vi "Edit_Channel_Panel.vi"(0 "All Channel names":string[](array[string])=["30-10-03:New:Channel new5"], 9 "Result files to read":path[](array[path])) -> (3 "New Values Out":string[](array[string])=["Test data5"], 4 "New Chs Out":string[](array[string])=["30-10-03:New:Channel new5"], 6 "Cancel Out":bool, 8 "Edit Raw Data Header Info Out":bool, 10 "Plotted rows only?":bool, 13 "Edit Raw data files?":bool, 14 "Raw data files in Orig Positions?":bool, 15 "Mode":T1)   [LabVIEW 2010]
uses:
  Plotter_Mode.ctl
panel:
  in  "Select channel names":bool
  in  "Cancel":bool
  in  "Edit Raw data files":i32(listbox)
  in  "Columns to Output":i32[](listbox)
  in  "Edit Type":i32(listbox)
  in  "OK Button":bool
  in  "Add values to:":i32(listbox)=1
  in  "New Values In":string[](array[string])=["Value"]
  in  "New Chs In":string[](array[string])=["Channel Name"]
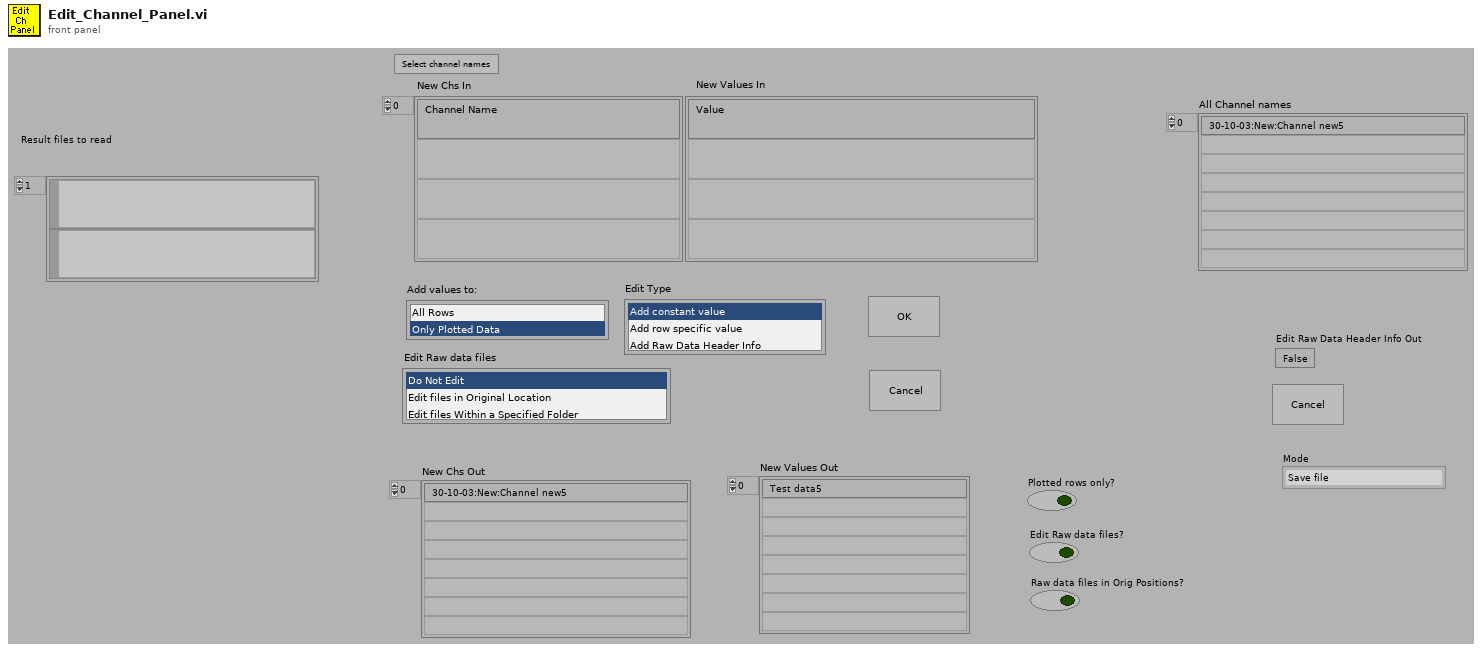
[diagram p1: front panel]
types:
  T1 = typedef "Plotter_Mode.ctl" = enum16{"Save file", "Delete unwanted rows", "Edit Values with constants", "Edit values per row", "Edit Raw Data file header", "Post Process Plotted Rows"}
  T2 = enum16{"Read Channels From File", "Read Channels from Server"}
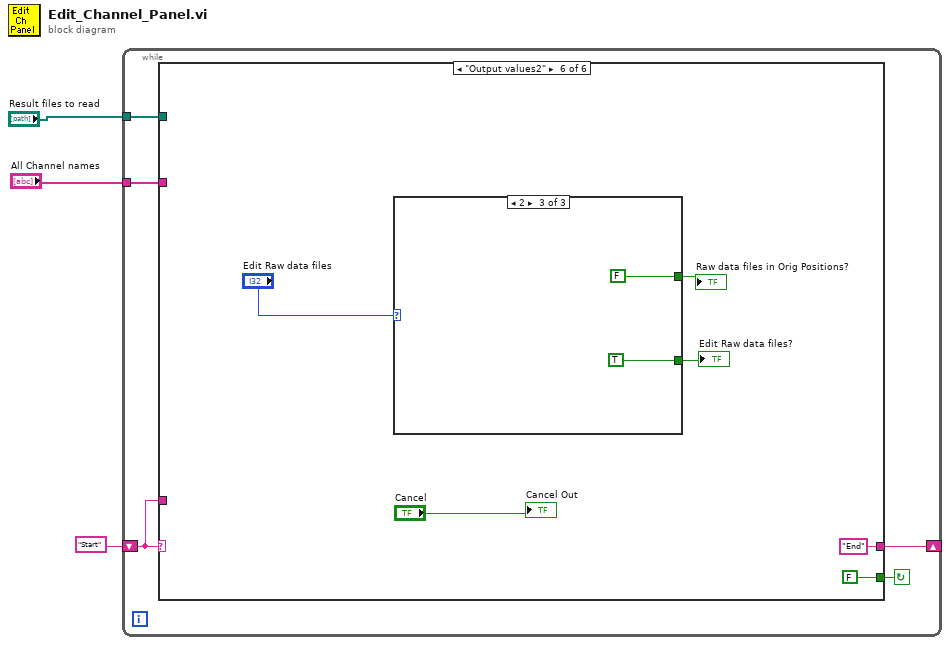
[diagram p0: block diagram]
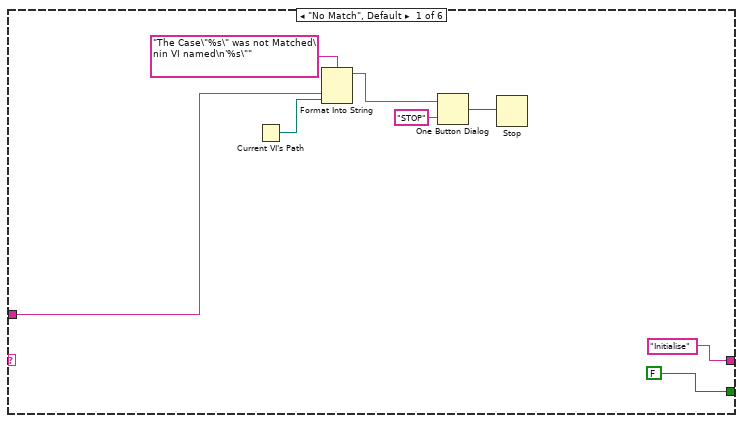
[diagram p2: hidden frame]
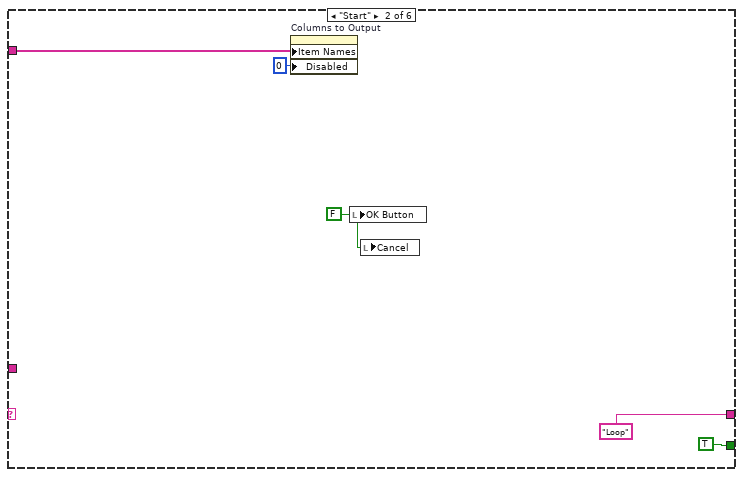
[diagram p3: hidden frame]
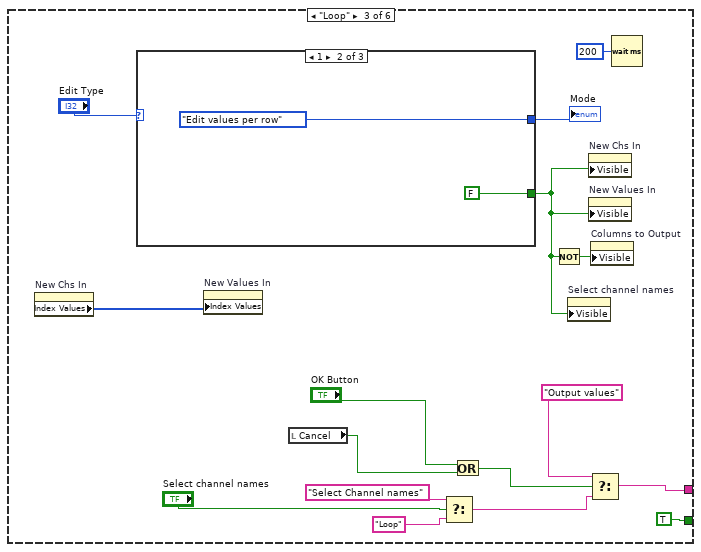
[diagram p4: hidden frame]
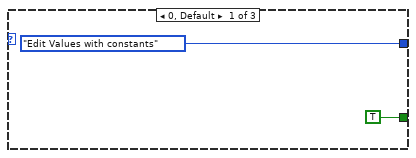
[diagram p5: hidden frame]
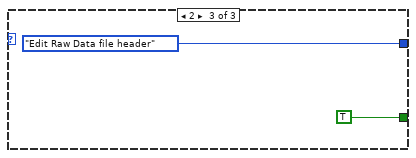
[diagram p6: hidden frame]
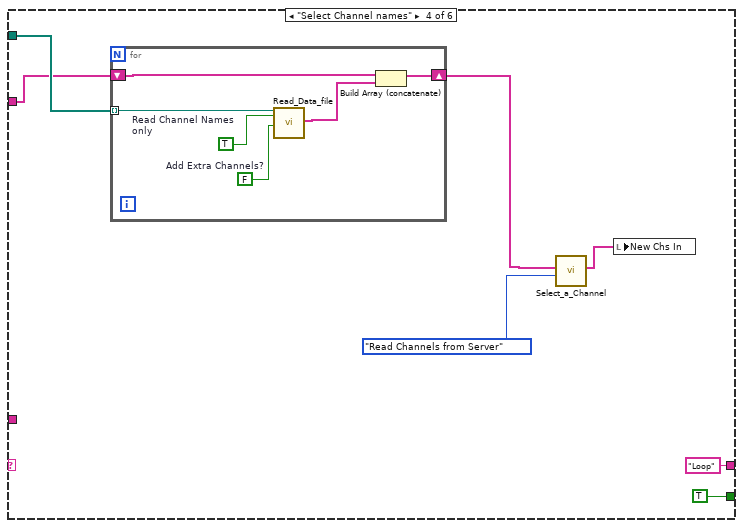
[diagram p7: hidden frame]
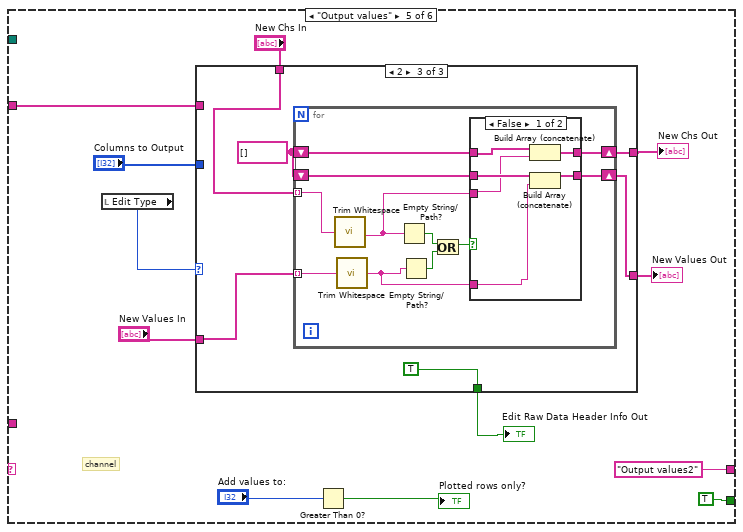
[diagram p8: hidden frame]
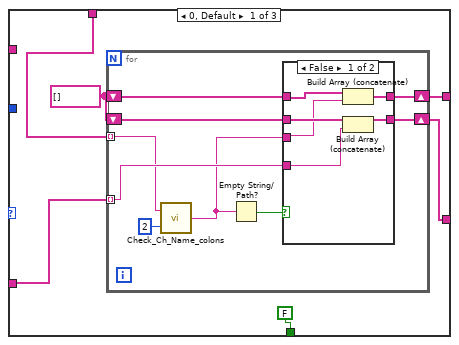
[diagram p9: hidden frame]
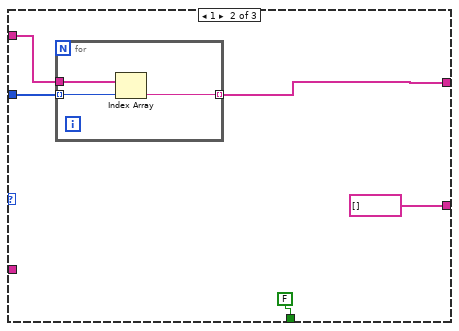
[diagram p11: hidden frame]
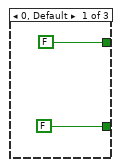
[diagram p13: hidden frame]
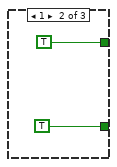
[diagram p14: hidden frame]
diagram:
  n1 = while {
    shift-left: "Start" -> [w6]
    shift-right: [w7] -> _
    tunnel: "All Channel names" -> [w5]
    tunnel: "Result files to read" -> [w4]
    stop <- w8 continue-if-true
    n2 = case shown="\"Output values2\"" w6 {
      tunnel: [FALSE TRUE TRUE TRUE TRUE FALSE] -> w8
      tunnel: ["Initialise" "Loop" w35 "Loop" "Output values2" "End"] -> w7
      tunnel: w6 -> [w11 _ _ _ _ _]
      tunnel: w5 -> [_ w19 _ w48 w58 _]
      tunnel: w4 -> [_ _ _ w49 _ _]
      frame "No Match", Default {
        n3 = Current VI's Path() -> (path=w10:path)
        n4 = Format Into String(format string="The Case\"%s\" was not Matched\nin VI named\n'%s\"" ("Format String"), w11, w10) -> (resulting string=w14:string)  [unwired: 2 in, 1 out]
        n5 = One Button Dialog(message=w14, button name ("OK")="STOP") -> (true=w12:bool)
        n6 = Stop(stop? (T)=w12) -> ()
      }
      frame "Start" {
        w17 = FALSE ("OK Button")
        n7 = property on="Columns to Output" class="LstBox (strict)"("Item Names"=w19, "Disabled"=u8 0) -> ()  [unwired: 2 in, 2 out]
        n8 = local write "OK Button"(w17) -> ()
        n9 = local write "Cancel"(w17) -> ()
      }
      frame "Loop" {
        n10 = property on="New Chs In" class="Arr (strict)"() -> ("Index Values"=w25:u32[])  [unwired: 2 in, 2 out]
        n11 = case shown="1" "Edit Type" {
          tunnel: [Plotter_Mode."Edit Values with constants" ("Mode") Plotter_Mode."Edit values per row" ("Mode") Plotter_Mode."Edit Raw Data file header" ("Mode")] -> w33
          tunnel: [TRUE FALSE TRUE] -> w22
          frame 0, Default {
          }
          frame 1 {
          }
          frame 2 {
          }
        }
        "Mode" <- w33
        n12 = property on="New Values In" class="Arr (strict)"("Index Values"=w25) -> ()  [unwired: 2 in, 2 out]
        n13 = local read "Cancel"() -> (w31:bool)
        n14 = Select(t="Select Channel names", s="Select channel names", f="Loop") -> (s? t:f=w24:string)
        n15 = Or(x="OK Button", y=w31) -> (x .or. y?=w29:bool)
        n16 = Not(x=w22) -> (.not. x?=w32:bool)
        n17 = property on="Select channel names" class="Bool"("Visible"=w22) -> ()  [unwired: 2 in, 2 out]
        n18 = property on="New Chs In" class="Arr (strict)"("Visible"=w22) -> ()  [unwired: 2 in, 2 out]
        n19 = property on="New Values In" class="Arr (strict)"("Visible"=w22) -> ()  [unwired: 2 in, 2 out]
        n20 = Select(t="Output values", s=w29, f=w24) -> (s? t:f=w35:string)
        n21 = property on="Columns to Output" class="LstBox (strict)"("Visible"=w32) -> ()  [unwired: 2 in, 2 out]
        n22 = Wait (ms)(milliseconds to wait=u32 200) -> ()  [unwired: 1 out]
      }
      frame "Select Channel names" {
        n23 = for {
          shift-right: [w53] -> w47
          shift-left: w48 -> [w51]
          tunnel: w49 -> [w56] mode=indexing
          w54 = FALSE  # Add Extra Channels?
          w55 = TRUE  # Read Channel Names only
          n24 = call "Read_Data_file.vi"("Results file"=w56, "Read Channel Names only"=w55, "Add Extra Channels?"=w54) -> ("Ch names Out"=w52:string[])  [unwired: 2 in, 14 out]
          n25 = Build Array (concatenate)(w51, w52) -> (w53:string[])
        }
        n26 = call "Select_a_Channel.vi"("Mode"=T2."Read Channels from Server", "Extra channel names"=w47) -> ("Selected Channel Names"=w46:string[])  [unwired: 1 in, 5 out]
        n27 = local write "New Chs In"(w46) -> ()
      }
      frame "Output values" {
        # "channel"
        n28 = local read "Edit Type"() -> (w64:i32)
        n29 = case shown="2" w64 {
          tunnel: "New Values In" -> [w72 _ w103]
          tunnel: [w71 string[] [] w102] -> w62
          tunnel: "New Chs In" -> [w73 _ w104]
          tunnel: [w70 w94 w101] -> w60
          tunnel: "Columns to Output" -> [_ w96 _]
          tunnel: w58 -> [_ w95 _]
          tunnel: [FALSE FALSE TRUE] -> w57
          frame 0, Default {
            w74 = string[] []
            n30 = for {
              tunnel: w72 -> [w79] mode=indexing
              shift-right: [w80] -> w70
              shift-left: w74 -> [w83]
              shift-right: [w82] -> w71
              shift-left: w74 -> [w81]
              tunnel: w73 -> [w78] mode=indexing
              n31 = call "Check_Ch_Name_colons.vi"("No of Colons"=2, "Ch Name in"=w78) -> ("Ch Name out"=w77:string)
              n32 = Empty String/Path?(string/path=w77) -> (empty?=w76:bool)
              n33 = case shown="False" w76 {
                tunnel: [w86 w91] -> w80
                tunnel: w83 -> [w89 w91]
                tunnel: [w87 w90] -> w82
                tunnel: w81 -> [w88 w90]
                tunnel: w79 -> [w84 _]
                tunnel: w77 -> [w85 _]
                frame False {
                  n34 = Build Array (concatenate)(w89, w85) -> (w86:string[])
                  n35 = Build Array (concatenate)(w88, w84) -> (w87:string[])
                }
                frame True {
                }
              }
            }
          }
          frame 1 {
            n36 = for {
              tunnel: w96 -> [w99] mode=indexing
              tunnel: w95 -> [w98]
              tunnel: [w97] -> w94 mode=indexing
              n37 = Index Array(array=w98, index=w99) -> (element=w97:string)
            }
          }
          frame 2 {
            w105 = string[] []
            n38 = for {
              tunnel: w103 -> [w111] mode=indexing
              shift-right: [w113] -> w101
              shift-left: w105 -> [w116]
              shift-right: [w115] -> w102
              shift-left: w105 -> [w114]
              tunnel: w104 -> [w112] mode=indexing
              n39 = call <vilib>:"Trim Whitespace.vi"("string"=w112) -> ("trimmed string"=w107:string)  [unwired: 1 in]
              n40 = call <vilib>:"Trim Whitespace.vi"("string"=w111) -> ("trimmed string"=w106:string)  [unwired: 1 in]
              n41 = Empty String/Path?(string/path=w107) -> (empty?=w109:bool)
              n42 = Empty String/Path?(string/path=w106) -> (empty?=w110:bool)
              n43 = Or(x=w109, y=w110) -> (x .or. y?=w108:bool)
              n44 = case shown="False" w108 {
                tunnel: [w119 w124] -> w113
                tunnel: w116 -> [w122 w124]
                tunnel: [w120 w123] -> w115
                tunnel: w114 -> [w121 w123]
                tunnel: w107 -> [w118 _]
                tunnel: w106 -> [w117 _]
                frame False {
                  n45 = Build Array (concatenate)(w122, w118) -> (w119:string[])
                  n46 = Build Array (concatenate)(w121, w117) -> (w120:string[])
                }
                frame True {
                }
              }
            }
          }
        }
        "New Values Out" <- w62
        "New Chs Out" <- w60
        "Edit Raw Data Header Info Out" <- w57
        n47 = Greater Than 0?(x="Add values to:") -> (x > 0?=→"Plotted rows only?":bool)
      }
      frame "Output values2" {
        n48 = case shown="2" "Edit Raw data files" {
          tunnel: [FALSE TRUE TRUE] -> w127
          tunnel: [FALSE TRUE FALSE] -> w126
          frame 0, Default {
          }
          frame 1 {
          }
          frame 2 {
          }
        }
        "Edit Raw data files?" <- w127
        "Raw data files in Orig Positions?" <- w126
        "Cancel Out" <- "Cancel"
      }
    }
  }
